vi "Set Default Trigger.vi"(7 "Trigger Direction":T2, 8 "error in (no error)":errorcluster, 10 "Default Trigger":T1, 11 "Item Ref in":T3 format="%.0x") -> (0 "error out":errorcluster, 3 "Item Ref out":T3 format="%.0x")   [LabVIEW 2015, in "Waveform Data Logger Shared.lvlib"]
uses:
  Waveform Data Logger Shared.lvlib
  <vilib>/NI Veristand/Custom Device API/Custom Device Item Ref.ctl
  Types/Trigger Direction.ctl
  Types/Default Trigger.ctl
  Globals/Property Strings.vi
  <vilib>/NI Veristand/Custom Device API/Set Item Property (Boolean).vi
  <vilib>/NI VeriStand/Custom Device API/Custom Device API.lvlib
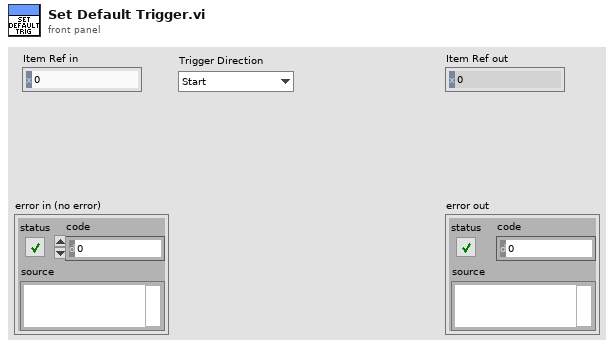
[diagram p1: front panel]
types:
  T1 = typedef "Waveform Data Logger Shared.lvlib/Default Trigger.ctl" = cluster{"Default State":bool}
  T2 = typedef "Waveform Data Logger Shared.lvlib/Trigger Direction.ctl" = enum16{"Start", "Stop"}
  T3 = typedef "Custom Device API.lvlib/Custom Device Item Ref.ctl" = u64
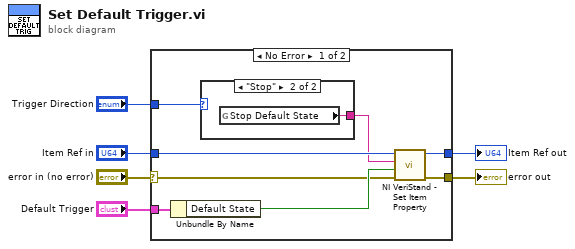
[diagram p0: block diagram]
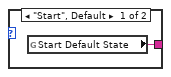
[diagram p2: hidden frame]
diagram:
  n1 = case shown="No Error" "error in (no error)" {
    selector: "error in (no error)" -> [w8 w17]
    tunnel: [w14 w18] -> w6
    tunnel: [w13 w17] -> w5
    tunnel: "Item Ref in" -> [w9 w18]
    tunnel: "Default Trigger" -> [w12 _]
    tunnel: "Trigger Direction" -> [w11 _]
    frame No Error {
      n2 = Unbundle By Name(w12) -> ("Default State"=w10:bool)
      n3 = case shown="\"Stop\"" w11 {
        tunnel: [w15 w16] -> w7
        frame "Start", Default {
          n4 = global read "Property Strings.vi" "Start Default State"() -> (w15:string)
        }
        frame "Stop" {
          n5 = global read "Property Strings.vi" "Stop Default State"() -> (w16:string)
        }
      }
      n6 = call-poly <vilib>:"NI VeriStand - Set Item Property.vi"("error in (no error)"=w8, "Value"=w10, "Property Name"=w7, "Item Ref in"=w9) -> ("error out"=w13:errorcluster, "Item Ref out"=w14:T3)  [unwired: 5 in, 1 out]
    }
    frame Error {
    }
  }
  "Item Ref out" <- w6
  "error out" <- w5
